vi "Set Detector.vi"(8 "error in (no error)":errorcluster, 10 "Muon Detector":refnum<class "Muon Detector.lvclass">, 11 "Detector Actor in":refnum<class "Detector Actor.lvclass">) -> (0 "error out":errorcluster, 3 "Detector Actor out":refnum<class "Detector Actor.lvclass">)   [LabVIEW 2019, in "Detector Actor.lvlib" / "Detector Actor.lvclass"]
uses:
  Detector Actor.lvclass
  Sensors/Detector/Muon Detector.lvclass
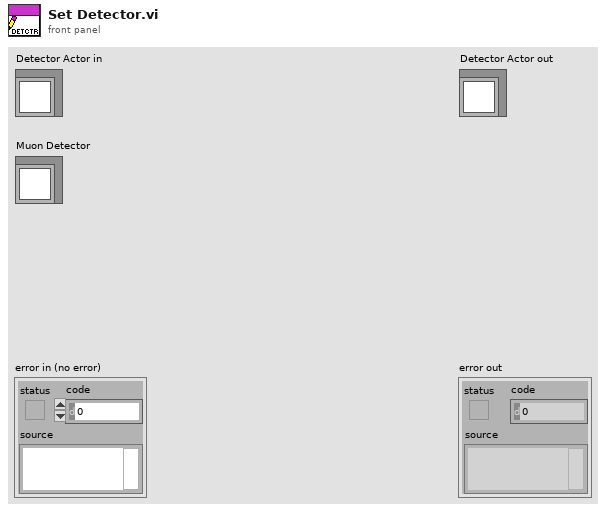
[diagram p1: front panel]
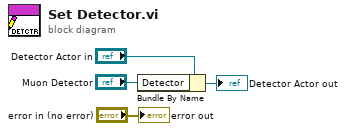
[diagram p0: block diagram]
diagram:
  n1 = Bundle By Name(cluster="Detector Actor in", "Detector"="Muon Detector") -> (→"Detector Actor out":refnum<class "Detector Actor.lvclass">)
  "error out" <- "error in (no error)"
